vi "Launch Plot.vi"(6 "Plot group":string, 8 "error in (no error)":errorcluster, 9 "Plot type":T1, 10 "File Path Control":path, 11 "Application Controller in":refnum<class "Application Controller.lvclass">) -> (0 "error out":errorcluster, 2 "Nested Actor's Enqueuer":refnum<class "Message Enqueuer.lvclass">, 3 "Application Controller out":refnum<class "Application Controller.lvclass">)   [LabVIEW 2016, in "Application Controller.lvclass"]
uses:
  Application Controller.lvclass
  Plots/Plot types.ctl
  <vilib>/ActorFramework/Message Enqueuer/Message Enqueuer.lvclass
  Plots/XY WFRM Plot/XY WFRM Plot.lvclass
  C:/github/LabActor/Plots/Plot/Plot.lvclass
  Plots/XY WFRM Plot/XY WFRM Plot.lvclass/XY WFRM Plot.ctl
  Plots/XY Plot/XY Plot.lvclass
  Application Controller.lvclass/Application Controller.ctl
  Plots/Plot Messages/Add file Msg/Add file Msg.lvclass/Add file Msg.ctl
  <vilib>/ActorFramework/Message Enqueuer/Message Enqueuer.lvclass/Message Enqueuer.ctl
  Plots/XY WFRM Plot/Write Plot type.vi
  <vilib>/ActorFramework/Message Enqueuer/Enqueue.vi
  Plots/Plot/Plot.lvclass
  C:/github/LabActor/Template Module/Template Module.lvclass
  Plots/Plot Messages/Add file Msg/Add file Msg.lvclass
  C:/Program Files/National Instruments/LabVIEW 2016/vi.lib/ActorFramework/Message/Message.lvclass
  Template Module Messages/Open Front Panel Msg/Open Front Panel Msg.lvclass
  <vilib>/ActorFramework/Message Priority Queue/Priority Enqueue.vi
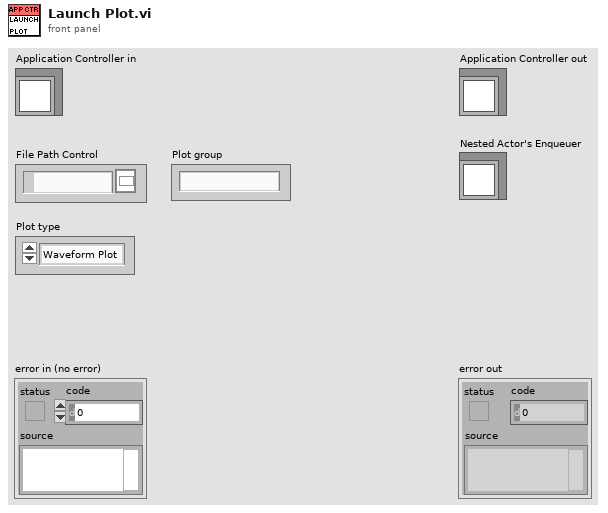
[diagram p1: front panel]
types:
  T1 = typedef "Plot types.ctl" = enum16{"Waveform Plot", "XY Plot", "Full XY"}
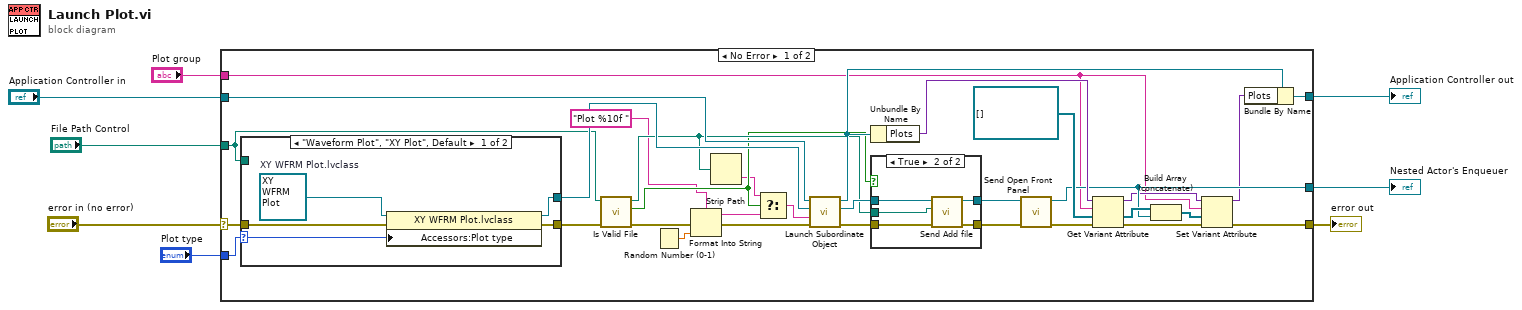
[diagram p0: block diagram]
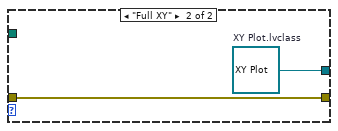
[diagram p3: hidden frame]
diagram:
  n1 = case shown="No Error" "error in (no error)" {
    selector: "error in (no error)" -> [w39 w56]
    tunnel: [w9 w56] -> w7
    tunnel: [w20 w55] -> w5
    tunnel: "Application Controller in" -> [w40 w55]
    tunnel: "File Path Control" -> [w33 _]
    tunnel: "Plot type" -> [w21 _]
    tunnel: [w16 _] -> w2
    tunnel: "Plot group" -> [w11 _]
    frame No Error {
      n2 = case shown="\"Waveform Plot\", \"XY Plot\", Default" w21 {
        selector: w21 -> [w48 _]
        tunnel: [w50 w54] -> w38
        tunnel: w33 -> [_ _]
        tunnel: [w49 w53] -> w32
        tunnel: w39 -> [w51 w53]
        frame "Waveform Plot", "XY Plot", Default {
          w52 = refnum<class "XY WFRM Plot.lvclass"> refnum  # XY WFRM Plot.lvclass
          n3 = property class="XY WFRM Plot.lvclass"(reference=w52, error in=w51, "Accessors:Plot type"=w48) -> (reference out=w50:refnum<class "XY WFRM Plot.lvclass">, error out=w49:errorcluster)
        }
        frame "Full XY" {
          w54 = refnum<class "XY Plot.lvclass"> refnum  # XY Plot.lvclass
        }
      }
      n4 = call "Is Valid File.vi"("Error In"=w32, "File"=w33) -> ("Error Out"=w22:errorcluster, "Valid file"=w29:bool, "File out"=w30:path)  [unwired: 7 in]
      n5 = Random Number (0-1)() -> (number: 0 to 1=w27:dbl)
      n6 = Format Into String(format string="Plot %10f ", error in=w22, w27) -> (resulting string=w25:string, error out=w23:errorcluster)  [unwired: 1 in]
      n7 = Strip Path(path=w30) -> (name=w28:string)  [unwired: 1 out]
      n8 = Select(t=w28, s=w29, f=w25) -> (s? t:f=w24:string)
      n9 = call-dynamic "Launch Subordinate Object.vi"("error in (no error)"=w23, "Name"=w24, "Subordinate Object"=w38, "Measure Object in"=w40) -> ("error out"=w31:errorcluster, "Nested Actor's Enqueuer"=w37:refnum<class "Message Enqueuer.lvclass">, "Measure Object out"=w34:refnum<class "Application Controller.lvclass">)  [unwired: 5 in]
      n10 = Unbundle By Name(w34) -> ("Plots"=w19:variant)
      n11 = case shown="True" w29 {
        tunnel: w37 -> [w42 w47]
        tunnel: [w42 w46] -> w36
        tunnel: [w41 w45] -> w35
        tunnel: w31 -> [w41 w44]
        tunnel: w30 -> [_ w43]
        frame False {
        }
        frame True {
          n12 = call "Send Add file.vi"("error in (no error)"=w44, "File Path Control"=w43, "Message Enqueuer"=w47) -> ("error out"=w45:errorcluster, "Message Enqueuer out"=w46:refnum<class "Message Enqueuer.lvclass">)  [unwired: 7 in]
        }
      }
      n13 = call "Send Open Front Panel.vi"("error in (no error)"=w35, "Message Enqueuer"=w36) -> ("error out"=w14:errorcluster, "Message Enqueuer out"=w16:refnum<class "Message Enqueuer.lvclass">)  [unwired: 8 in]
      n14 = Get Variant Attribute(Variant=w19, name=w11, default value (empty Variant)=refnum<class "Message Enqueuer.lvclass">[] [] ("Plot enqueuers"), error in=w14) -> (duplicate Variant=w15:variant, value=w17:refnum<class "Message Enqueuer.lvclass">[], error out=w13:errorcluster)  [unwired: 1 out]
      n15 = Build Array (concatenate)(w17, w16) -> (w12:refnum<class "Message Enqueuer.lvclass">[])
      n16 = Set Variant Attribute(Variant=w15, name=w11, value=w12, error in=w13) -> (Variant out=w10:variant, error out=w9:errorcluster)  [unwired: 1 out]
      n17 = Bundle By Name(cluster=w34, "Plots"=w10) -> (w20:refnum<class "Application Controller.lvclass">)
    }
    frame Error {
    }
  }
  "error out" <- w7
  "Application Controller out" <- w5
  "Nested Actor's Enqueuer" <- w2
